vi "module.vi"(10 "2D vector":dbl[](array[numeric])) -> (2 "Modulo":dbl)   [LabVIEW 2018, in "Utilities.lvclass"]
uses:
  Utilities.lvclass
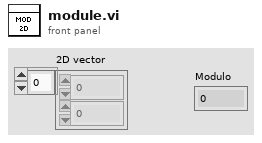
[diagram p1: front panel]
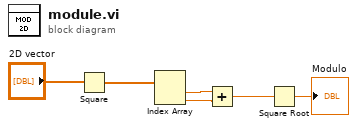
[diagram p0: block diagram]
diagram:
  n1 = Square(x="2D vector") -> (x^2=w6:dbl[])
  n2 = Index Array(array=w6) -> (element #1=w5:dbl, element #2=w4:dbl)  [unwired: 2 in]
  n3 = Add(x=w5, y=w4) -> (x+y=w2:dbl)
  n4 = Square Root(x=w2) -> (sqrt(x)=→"Modulo":dbl)
